vi "Pressure_Display&Log.vi"() -> ()   [LabVIEW 2016]
uses:
  <vilib>/express/express signal manip/GetorSetDDTAttributes/Shared VIs/TimeType.ctl
  <vilib>/express/express signal manip/GetorSetDDTAttributes/Shared VIs/XDimension.ctl
  <vilib>/NI/Modbus Library/API/Wrapper/Create Serial Master.vi
  <vilib>/express/express signal manip/GetorSetDDTAttributes/Shared VIs/TimeMode Enum to Boolean.vi
  <vilib>/express/express signal manip/GetorSetDDTAttributes/Shared VIs/XDimension Enum to String.vi
  <vilib>/express/express shared/transition.llb/Dynamic To Waveform Array.vi
  <vilib>/express/express signal manip/GetorSetDDTAttributes/Set DDT Attributes/SetT0.vi
  <vilib>/express/express shared/transition.llb/Waveform Array To Dynamic.vi
  <vilib>/express/express signal manip/GetorSetDDTAttributes/Set DDT Attributes/Set DDT Properties.xnode
  <vilib>/NI/Modbus Library/API/Master/Modbus Master.lvclass
  <vilib>/NI/Modbus Library/API/Wrapper/API Main.lvlib
  <vilib>/express/express signal manip/GetorSetDDTAttributes/Shared VIs/GetSetShared.lvlib
panel:
  in  "flow control (none)":u16(ring) items=["None", "XON/XOFF", "RTS/CTS", "XON/XOFF & RTS/CTS", "DTR/DSR", "XON/XOFF & DTR/DSR"]
  in  "parity (even)":u16(ring) items=["None", "Odd", "Even", "Mark", "Space"]
  in  "baud rate":u32=19200
  in  "VISA resource name":refnum<visa-resource-name>="COM11"
  out "Waveform Chart":dynamicdata(graph)
  out "Pirani  (mbar)":dbl
  out "LT":dbl format="%_3e"
  out "PREP":dbl format="%_3e"
  in  "stop":bool
  # "(mbar)"
  # "(mbar)"
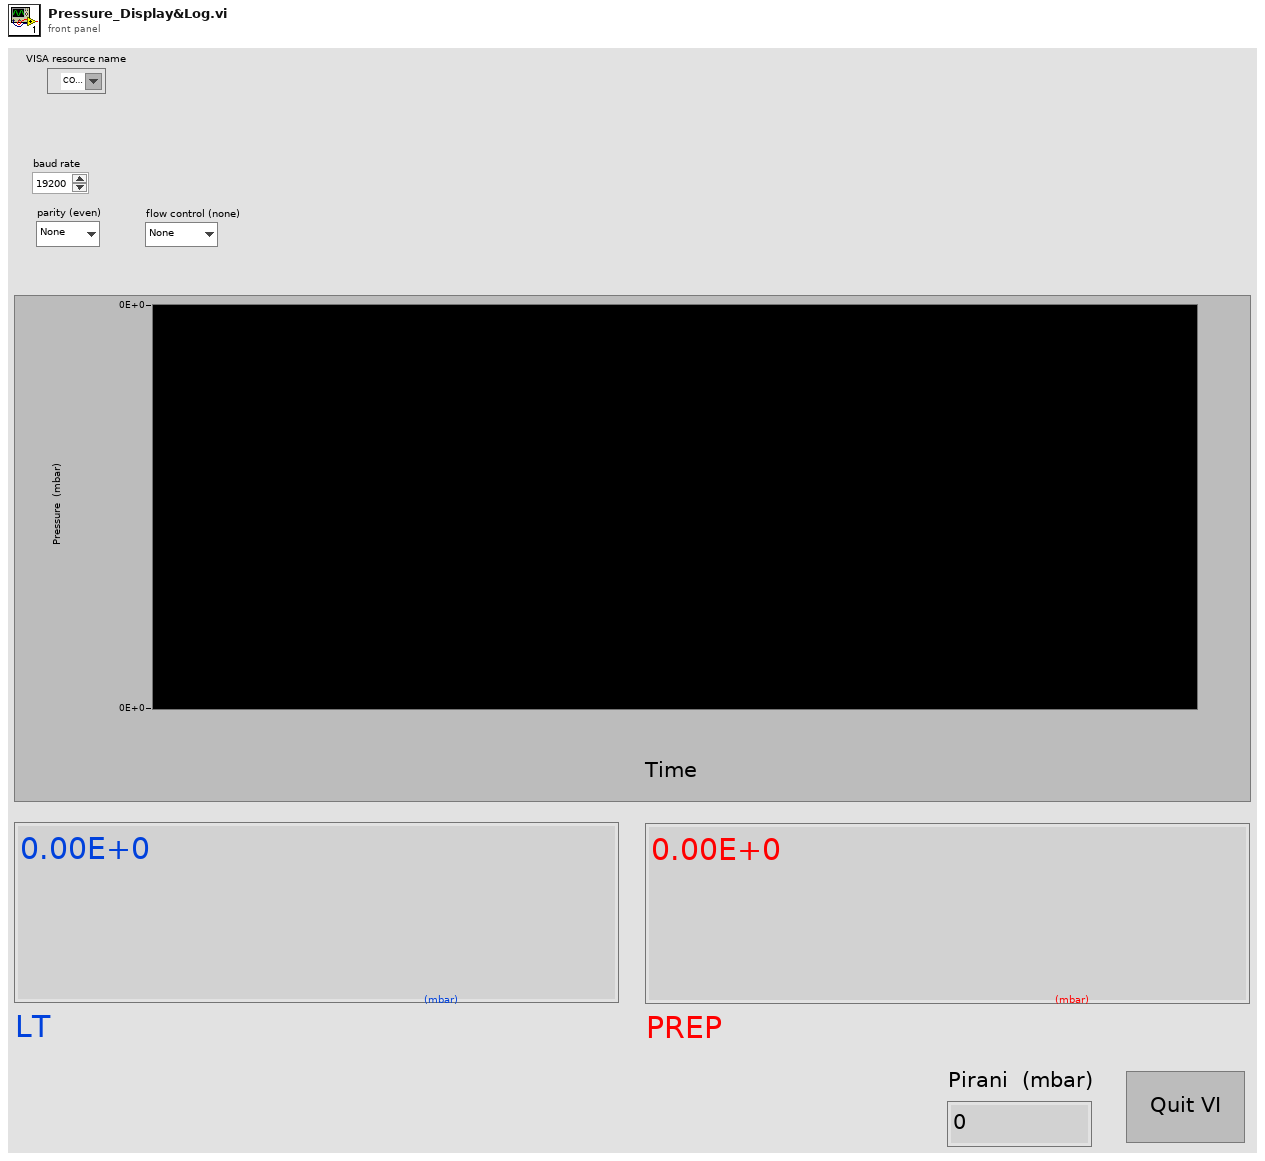
[diagram p1: front panel]
types:
  T1 = enum16{"open", "replace", "create", "open or create", "replace or create", "replace or create with confirmation"}
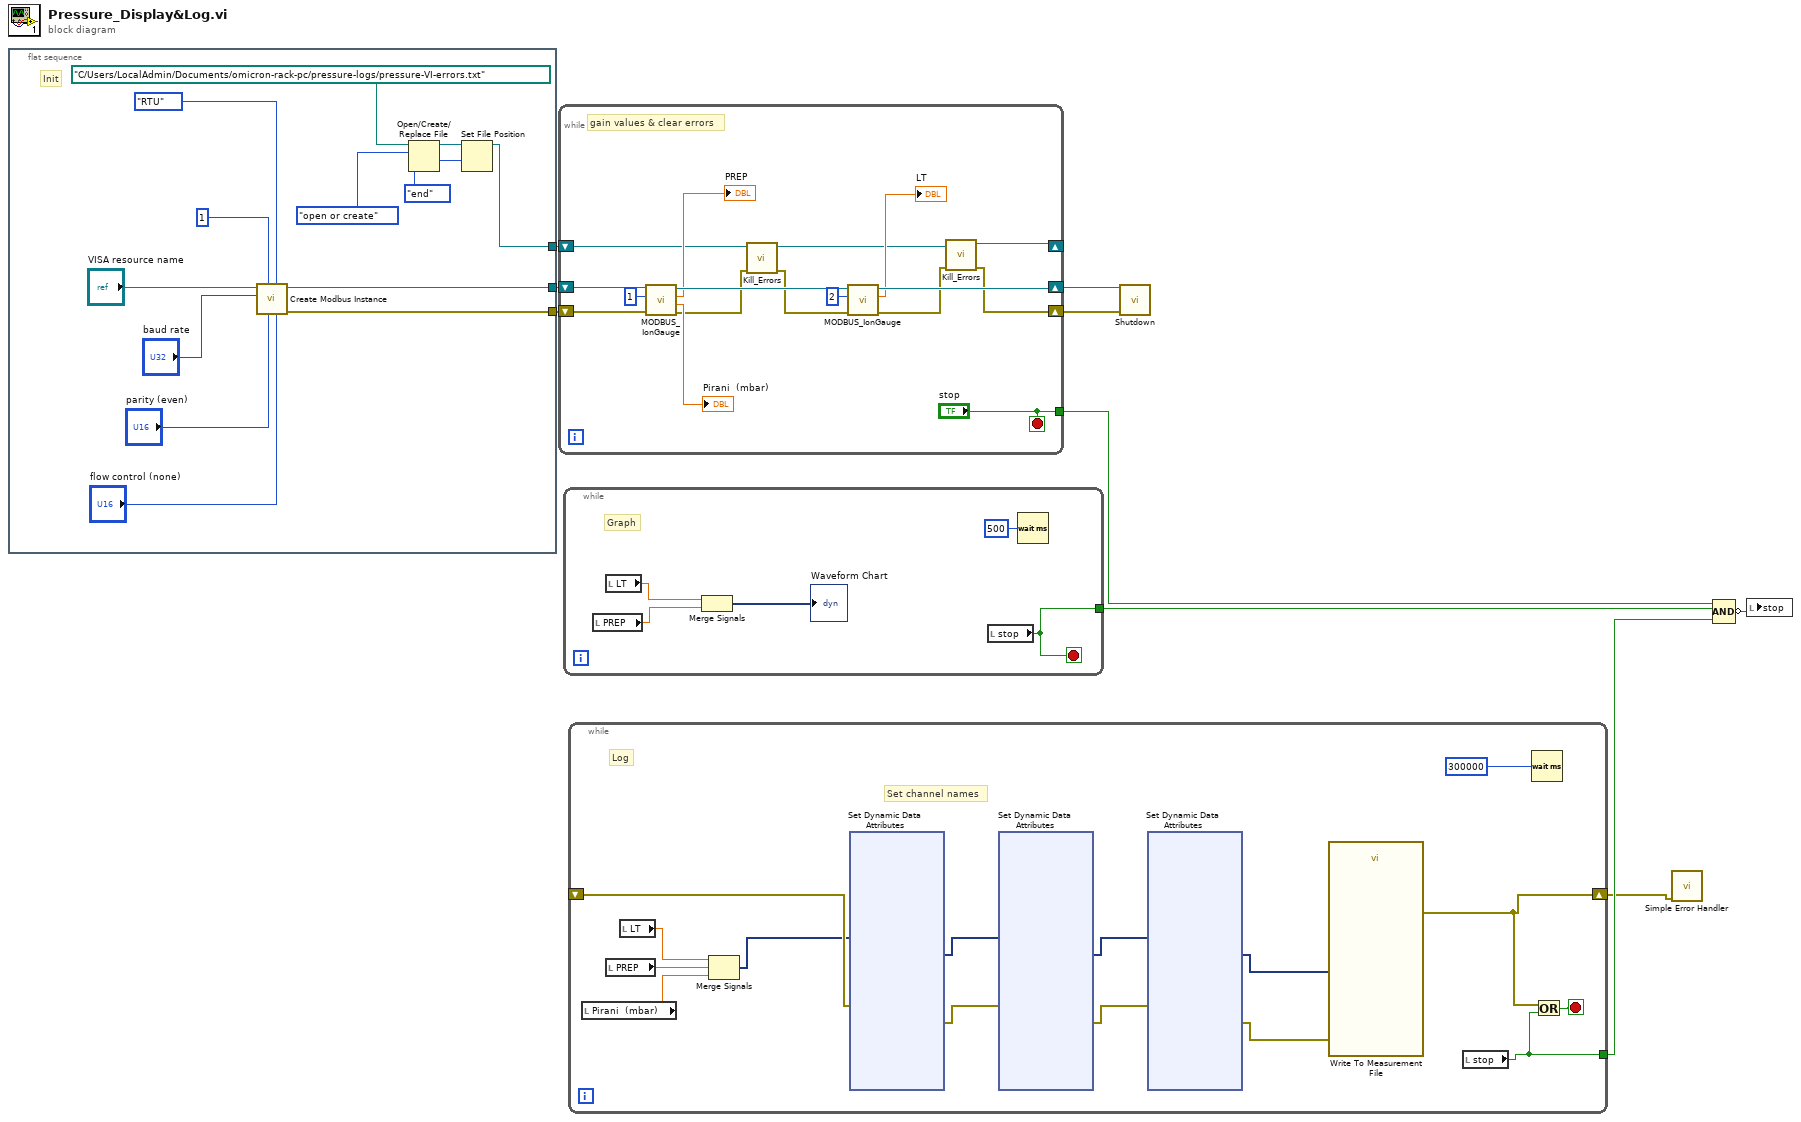
[diagram p0: block diagram]
diagram:
  n1 = flat-sequence {
    tunnel: [w17] -> w10
    tunnel: [w16] -> w9
    tunnel: [w12] -> w3
    frame #0 {
      # "Init"
      n2 = call-poly <vilib>:"Create Modbus Instance.vi"("flow control (none)"="flow control (none)", "serial type"=enum16{"RTU", "ASCII"}."RTU", "parity (even)"="parity (even)", "unit ID"=u8 1, "baud rate"="baud rate", "VISA resource name"="VISA resource name") -> ("error out"=w16:errorcluster, "serial master instance"=w17:refnum<class "Modbus Master.lvclass">)  [unwired: 4 in]
      n3 = Open/Create/Replace File(file path (use dialog)=path "C:/Users/LocalAdmin/Documents/omicron-rack-pc/pressure-logs/pressure-VI-errors.txt" ("Path"), operation (0:open)=T1."open or create") -> (refnum out=w13:refnum<file>)  [unwired: 4 in, 2 out]
      n4 = Set File Position(refnum=w13, from (0:start)=enum16{"start", "end", "current"}."end") -> (refnum out=w12:refnum<file>)  [unwired: 2 in, 1 out]
    }
  }
  n5 = while {
    tunnel: ["stop"] -> w7
    shift-right: [w36] -> w5
    shift-left: w10 -> [w39]
    shift-right: [w27] -> w4
    shift-left: w9 -> [w38]
    shift-right: [w24] -> _
    shift-left: w3 -> [w26]
    stop <- "stop" stop-if-true
    # "gain values & clear errors"
    n6 = call "MODBUS_IonGauge.vi"("error in"=w38, "unit ID"=u8 1, "Modbus instance in"=w39) -> ("error out"=w30:errorcluster, "Pirani"=→"Pirani  (mbar)":sgl, "Ion Gauge Pressure"=→"PREP":sgl, "Modbus instance out"=w37:refnum<class "Modbus Master.lvclass">)  [unwired: 5 in]
    n7 = call "Kill_Errors.vi"("error in (no error)"=w30, "refnum in"=w26) -> ("error out"=w29:errorcluster, "refnum"=w25:refnum<file>)  [unwired: 8 in]
    n8 = call "MODBUS_IonGauge.vi"("error in"=w29, "unit ID"=u8 2, "Modbus instance in"=w37) -> ("error out"=w28:errorcluster, "Ion Gauge Pressure"=→"LT":sgl, "Modbus instance out"=w36:refnum<class "Modbus Master.lvclass">)  [unwired: 5 in, 1 out]
    n9 = call "Kill_Errors.vi"("error in (no error)"=w28, "refnum in"=w25) -> ("error out"=w27:errorcluster, "refnum"=w24:refnum<file>)  [unwired: 8 in]
  }
  n10 = while {
    tunnel: [w43] -> w6
    stop <- w43 stop-if-true
    # "Graph"
    n11 = local read "PREP"() -> (w41:dbl)
    n12 = local read "LT"() -> (w42:dbl)
    n13 = Merge Signals(w42, w41) -> (→"Waveform Chart":dynamicdata)
    n14 = local read "stop"() -> (w43:bool)
    n15 = Wait (ms)(milliseconds to wait=u32 500) -> ()  [unwired: 1 out]
  }
  n16 = while {
    tunnel: [w48] -> w2
    shift-right: [w47] -> w1
    shift-left: _ -> [w56]
    stop <- w46 stop-if-true
    # "Set channel names"
    # "Log"
    n17 = local read "Pirani  (mbar)"() -> (w57:dbl)
    n18 = local read "PREP"() -> (w58:dbl)
    n19 = local read "LT"() -> (w59:dbl)
    n20 = Merge Signals(w59, w58, w57) -> (w52:dynamicdata)
    n21 = xnode "Set Dynamic Data Attributes"("Signals In"=w52, "error in"=w56) -> ("Signals Out"=w51:dynamicdata, "error out"=w55:errorcluster)  [unwired: 5 in]
    n22 = xnode "Set Dynamic Data Attributes"("Signals In"=w51, "error in"=w55) -> ("Signals Out"=w50:dynamicdata, "error out"=w54:errorcluster)  [unwired: 5 in]
    n23 = xnode "Set Dynamic Data Attributes"("Signals In"=w50, "error in"=w54) -> ("Signals Out"=w49:dynamicdata, "error out"=w53:errorcluster)  [unwired: 5 in]
    n24 = call "Write To Measurement File"("Signals"=w49, "error in (no error)"=w53) -> ("error out"=w47:errorcluster)  [unwired: 15 in, 2 out]
    n25 = local read "stop"() -> (w48:bool)
    n26 = Wait (ms)(milliseconds to wait=u32 300000) -> ()  [unwired: 1 out]
    n27 = Or(x=w47, y=w48) -> (x .or. y?=w46:bool)
  }
  n28 = call-dynamic "Shutdown.vi"("error in"=w4, "Modbus master in"=w5) -> ()  [unwired: 9 in, 1 out]
  n29 = call <vilib>:"Simple Error Handler.vi"("error in (no error)"=w1) -> ()  [unwired: 4 in, 5 out]
  n30 = Compound Arithmetic op=AND(w7, w6, w2) -> (invert w8:bool)
  n31 = local write "stop"(w8) -> ()
